vi "Write JSON Config.vi"(6 "Pretty Print?":bool, 8 "error in (no error)":errorcluster, 11 "AbsFunc_One Term_U16 in":refnum<class "AbsFunc_One Term_U16.lvclass">) -> (0 "error out":errorcluster, 2 "JSON":string, 3 "AbsFunc_One Term_U16 out":refnum<class "AbsFunc_One Term_U16.lvclass">)   [LabVIEW 2021, in "AbsFunc_One Term_U16.lvclass"]
uses:
  AbsFunc_One Term_U16.lvclass
  AbsFunc_One Term_U16.lvclass/AbsFunc_One Term_U16.ctl
  Abs_Types/Type/Abs_Type.lvclass
  Abs_Types/U16 Integer/Abs_U16 Integer.lvclass
  C:/Users/Tim/Documents/GitHub/LV_Abstract/Source/Abs_Types/U16 Integer/Abs_U16 Integer.lvclass
  C:/Users/Tim/Documents/GitHub/LV_Abstract/Source/Abs_Types/Integer/Abs_Integer.lvclass
  C:/Users/Tim/Documents/GitHub/LV_Abstract/Source/Abs_Types/Numeric/Abs_Numeric.lvclass
  C:/Users/Tim/Documents/GitHub/LV_Abstract/Source/Abs_Types/Value/Abs_Value.lvclass
  C:/Users/Tim/Documents/GitHub/LV_Abstract/Source/Abs_Types/Type/Abs_Type.lvclass
  C:/Users/Tim/Documents/GitHub/LV_Abstract/Source/Functions/Support/One Terminal/U16/AbsFunc_One Term_U16.lvclass
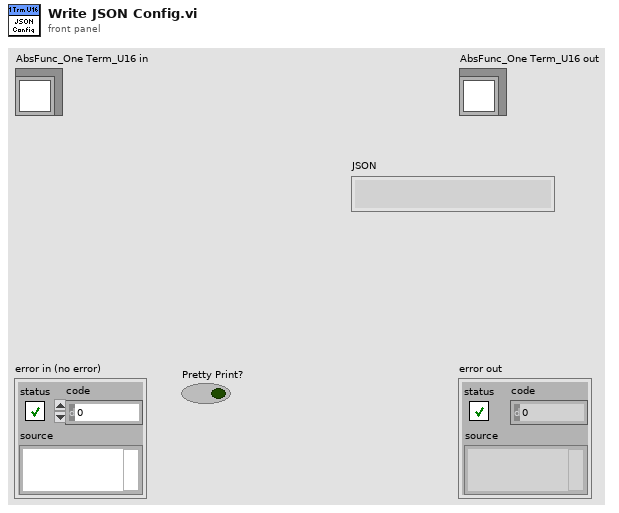
[diagram p1: front panel]
types:
  T1 = typedef "AbsFunc_One Term_U16.lvclass/Abstract Type.ctl" = refnum<class "Abs_U16 Integer.lvclass">
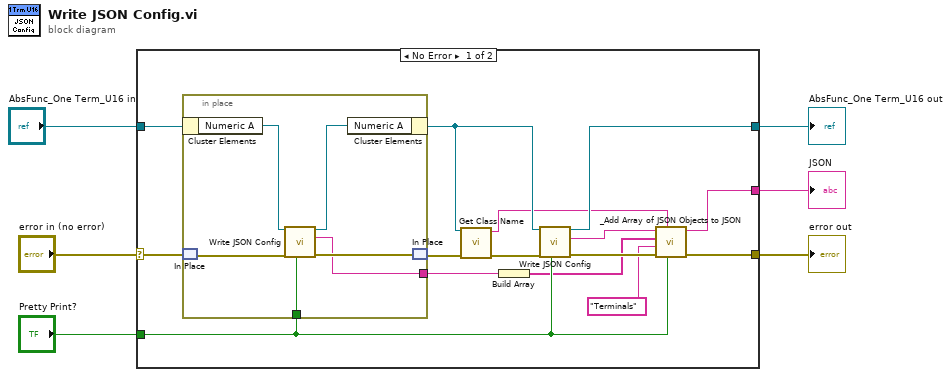
[diagram p0: block diagram]
diagram:
  n1 = case shown="No Error" "error in (no error)" {
    selector: "error in (no error)" -> [w17 w29]
    tunnel: "AbsFunc_One Term_U16 in" -> [w21 w28]
    tunnel: [w20 w28] -> w3
    tunnel: [w13 _] -> w4
    tunnel: [w12 w29] -> w5
    tunnel: "Pretty Print?" -> [w11 _]
    frame No Error {
      n2 = in-place {
        in-place-border: w11 -> [w26]
        in-place-border: [w24] -> w19
        n3 = in-place-cluster #1(w21) -> ("Numeric A"=w23:T1)
        n4 = in-place-match #2(w17) -> (w27:errorcluster)
        n5 = call-dynamic "Write JSON Config.vi"("Pretty Print?"=w26, "error in (no error)"=w27, "Abs_Type in"=w23) -> ("error out"=w25:errorcluster, "JSON"=w24:string, "Abs_Type out"=w22:T1)  [unwired: 6 in]
        n6 = in-place-cluster #1("Numeric A"=w22) -> (w15:refnum<class "AbsFunc_One Term_U16.lvclass">)
        n7 = in-place-match #2(w25) -> (w18:errorcluster)
      }
      n8 = call "Get Class Name.vi"("error in (no error)"=w18, "Abs_Type in"=w15) -> ("error out"=w16:errorcluster, "class name"=w10:string)  [unwired: 8 in]
      n9 = Build Array(w19) -> (w8:string[])
      n10 = call-parent "Write JSON Config.vi"("Pretty Print?"=w11, "error in (no error)"=w16, "Abs_Type in"=w15) -> ("error out"=w14:errorcluster, "JSON"=w9:string, "Abs_Type out"=w20:refnum<class "AbsFunc_One Term_U16.lvclass">)  [unwired: 6 in]
      n11 = call "_Add Array of JSON Objects to JSON.vi"("Pretty Print?"=w11, "JSON Object Name"=w10, "error in (no error)"=w14, "JSON Array Name"="Terminals", "JSON Objects"=w8, "JSON"=w9) -> ("error out"=w12:errorcluster, "<JSON>"=w13:string)  [unwired: 4 in]
    }
    frame Error {
    }
  }
  "error out" <- w5
  "AbsFunc_One Term_U16 out" <- w3
  "JSON" <- w4
